vi "Function.vi"(8 "Error In":errorcluster) -> (0 "Error Out":errorcluster)   [LabVIEW 2019, in "Library B.lvlib"]
uses:
  Library B.lvlib
  obj/TargetsDifferentCompilePPLHierarchy/Windows (x86)/Libraries/Library A.lvlibp
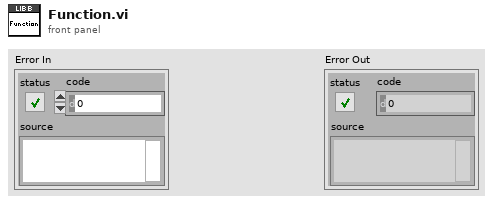
[diagram p1: front panel]
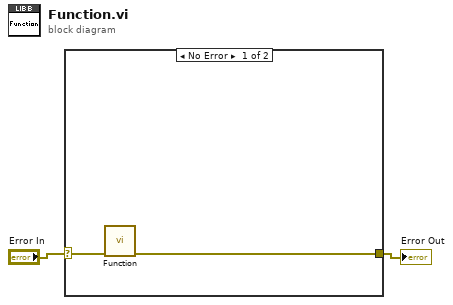
[diagram p0: block diagram]
diagram:
  n1 = case shown="No Error" "Error In" {
    selector: "Error In" -> [w4 w5]
    tunnel: [w3 w5] -> w1
    frame No Error {
      n2 = call "Function.vi"("Error In"=w4) -> ("Error Out"=w3:errorcluster)  [unwired: 10 in]
    }
    frame Error {
    }
  }
  "Error Out" <- w1
